vi "uTTA_Calibration_ADC.vi"(6 "AR488_in":refnum<visa-resource-name>, 7 "CommandQueue":refnum<queue>, 8 "error in":errorcluster, 9 "FunctionGen_In":refnum<visa-resource-name>, 10 "DataQueue":refnum<queue>, 11 "TDMS_FileIn":refnum<k34>) -> (0 "error out":errorcluster, 1 "FunctionGen_Out":refnum<visa-resource-name>, 2 "abort":bool, 3 "TDMS_FileOut":refnum<k34>, 4 "AR488_out":refnum<visa-resource-name>)   [LabVIEW 2021]
uses:
  <vilib>/Utility/miscctls.llb/LVPointTypeDef.ctl
  <vilib>/Analysis/6fits.llb/Curve Fitting Criteria.ctl
  eb1c96f3-5bac-4f55-aaa1-37eec1307aa8.vi
  <vilib>/Analysis/NI_AALPro.lvlib
panel:
  out "Voffs Zero Position":dbl
  out "DAC offset":dbl format="%#_6pV"
  out "DAC Residue":dbl caption="Residue" format="%.3p"
  out "DAC slope":dbl format="%#_4pV/Digit"
  in  "START":bool
  out "ADC_Values":dbl[](array[numeric]) format="%#.2g"
  out "ADC_Variance":dbl[](array[numeric]) format="%#.2g"
  out "ADC offset":dbl format="%#_6pV"
  out "ADC lin. res":dbl caption="Residue" format="%.3p"
  out "ADC slope":dbl format="%#_4pV/Digit"
  out "Ref. Setting":u32
  out "ADC Cal.":T1(graph)
  out "PGA setting":u32
  out "Calibration of Channel":u32
  in  "DAC Increments":u32=1000 caption="DAC Voltage\nIncrement" min=1 max=10000 step=1 format="%.3d Counts/Step"
  out "Status":string="Exit"
  in  "abort":bool
  # "1. Connect the function generator with a 50Ohm Terminator and a BNC Y-Adaptor to the input of the uTTA.\n2. Connect a ground lead to the outer Conductor of the BNC line to provide propper grounding\n3. Start the calibration"
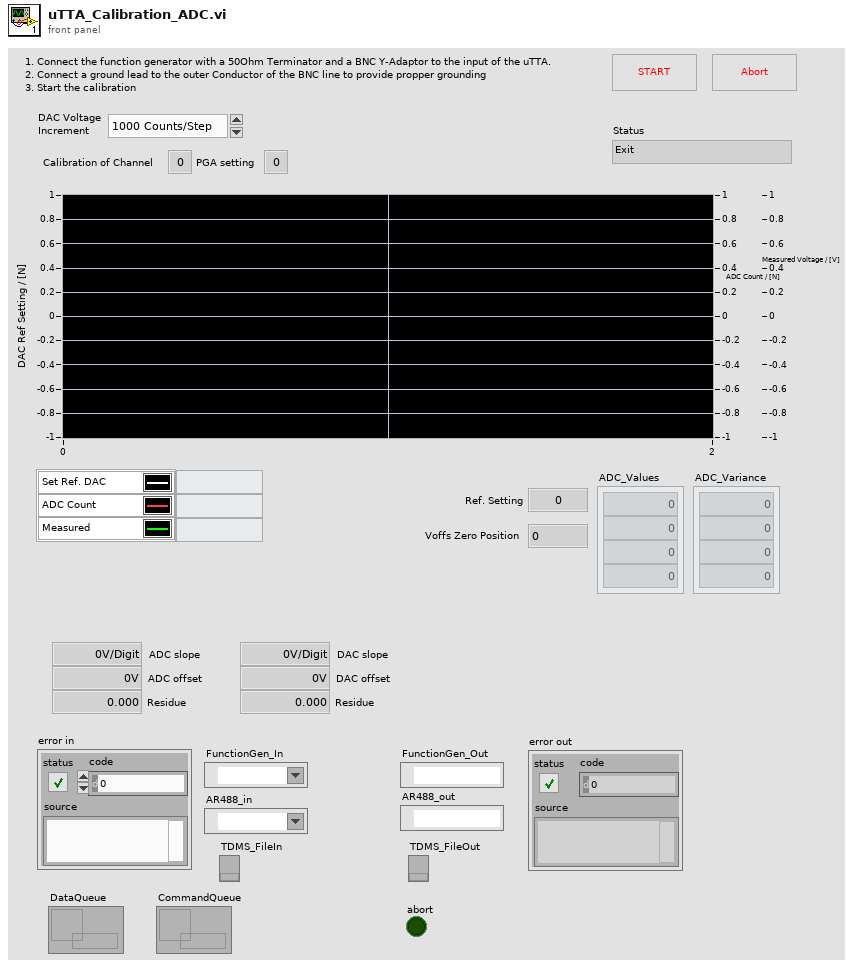
[diagram p1: front panel]
types:
  T1 = cluster{"Ref_Voltage":u32, "mean":dbl, "mean":dbl}
  T2 = typedef "LVPointTypeDef.ctl" = cluster{"Horizontal":i16, "Vertical":i16}
  T3 = cluster{"Ref_Voltage":u32, "mean":dbl, "mean":dbl}[]
  T4 = typedef "NI_AALPro.lvlib/Curve Fitting Criteria.ctl" = u16
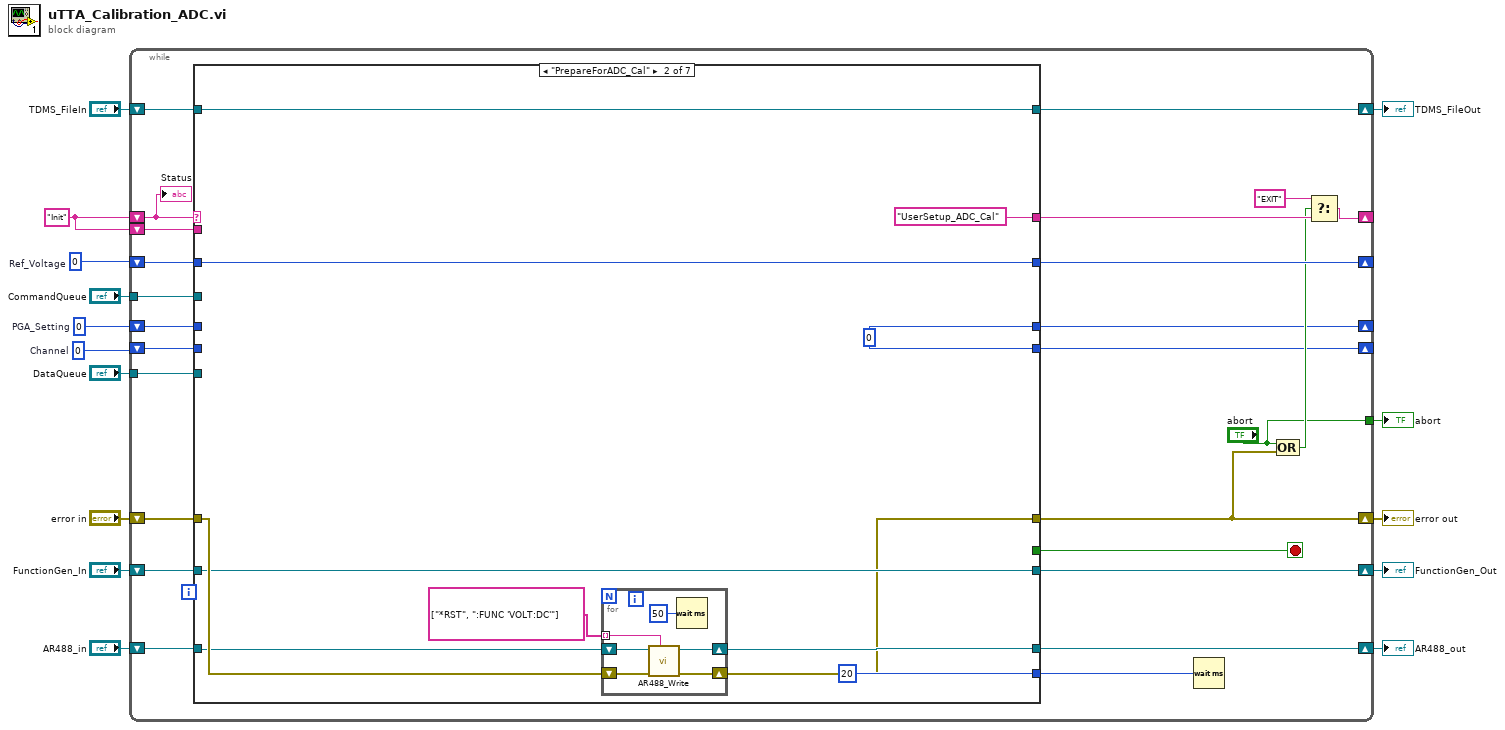
[diagram p0: block diagram]
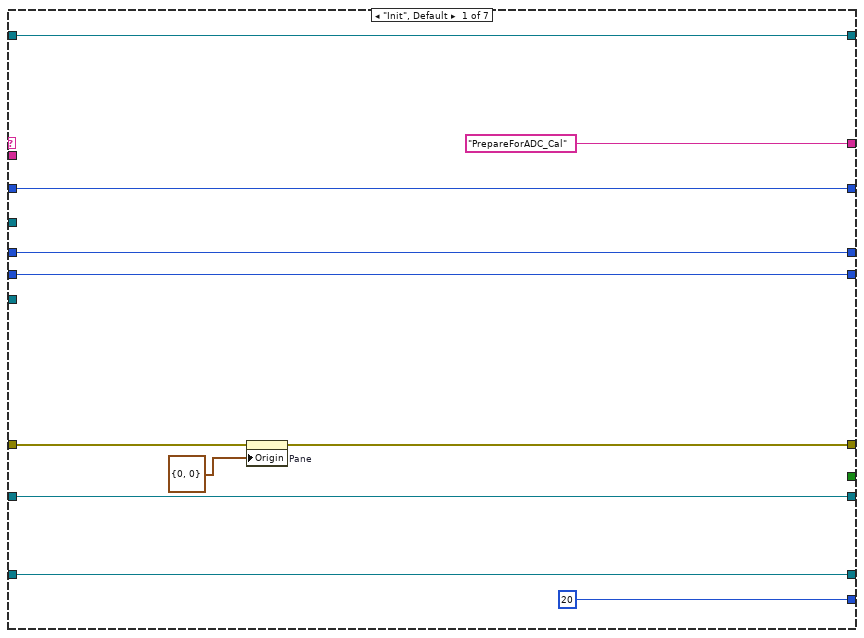
[diagram p2: hidden frame]
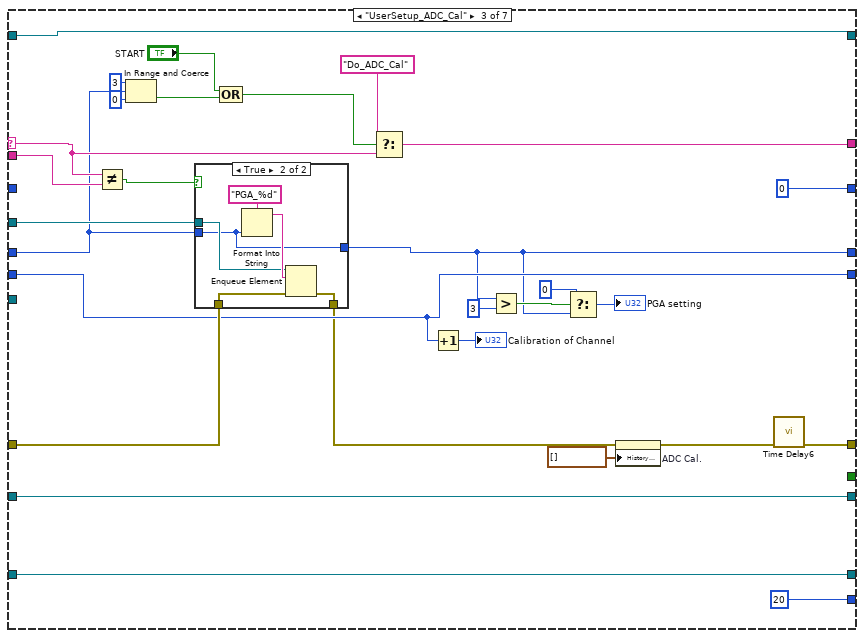
[diagram p3: hidden frame]
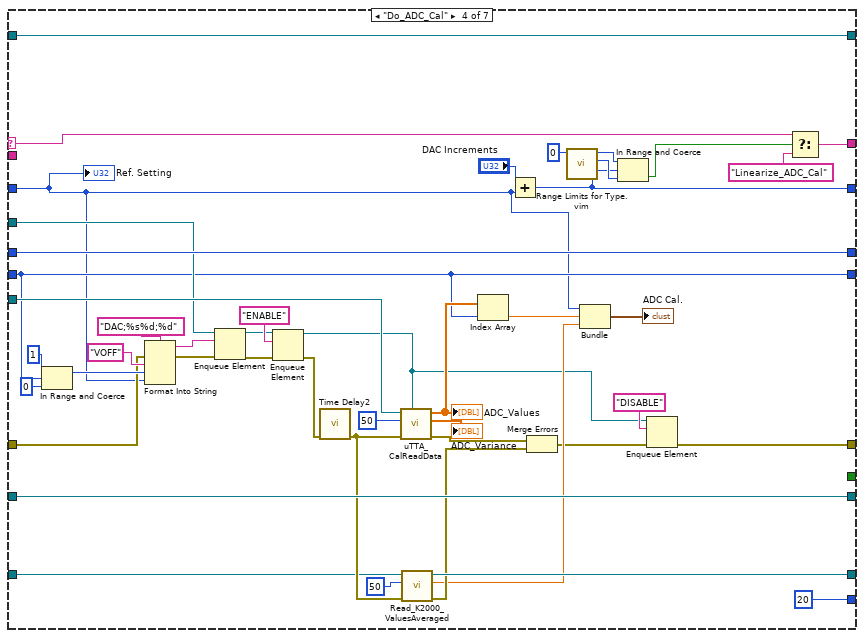
[diagram p5: hidden frame]
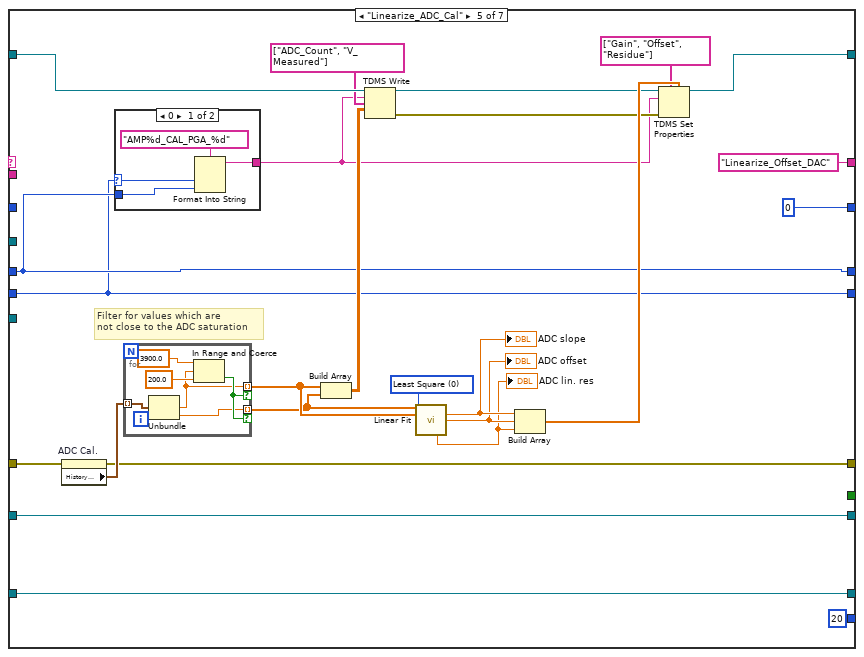
[diagram p6: hidden frame]
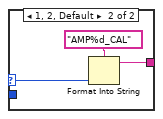
[diagram p7: hidden frame]
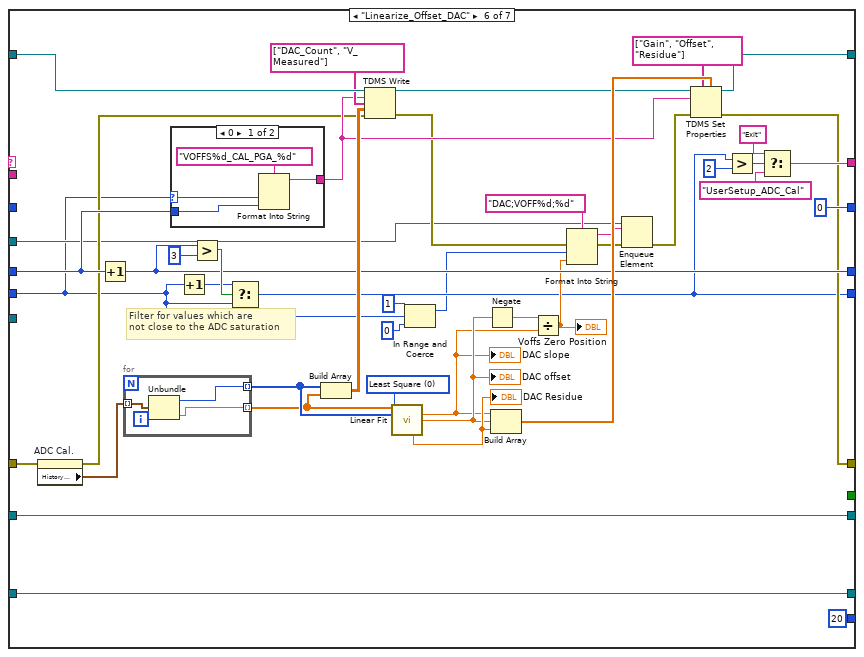
[diagram p8: hidden frame]
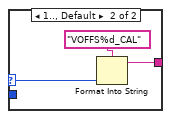
[diagram p9: hidden frame]
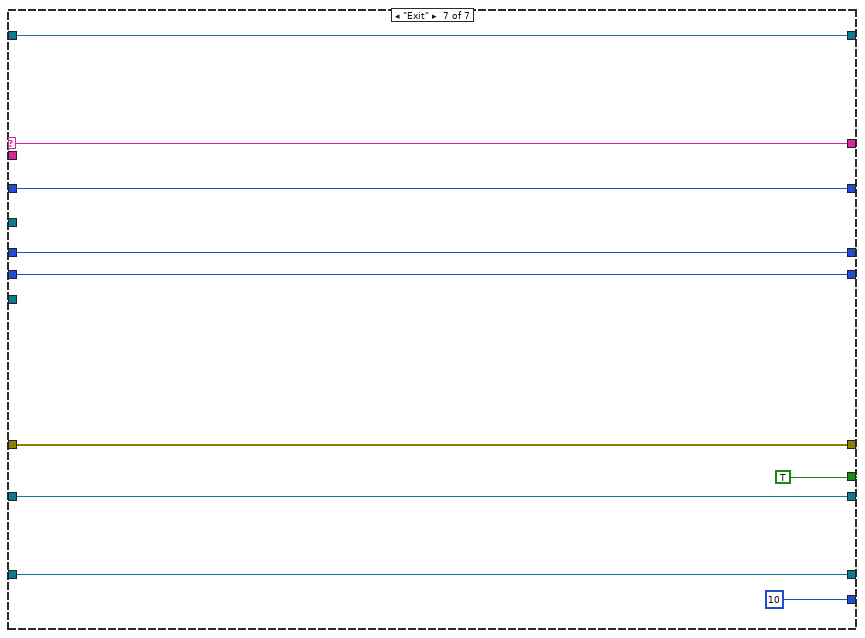
[diagram p10: hidden frame]
diagram:
  w11 = 0  # Channel
  w12 = 0  # PGA_Setting
  w14 = u32 0  # Ref_Voltage
  w13 = "Init"
  n1 = while {
    shift-right: [w27] -> _
    shift-left: w13 -> [w38]
    shift-right: [w25] -> w15
    shift-left: "error in" -> [w40]
    shift-right: [w36] -> w3
    shift-left: "FunctionGen_In" -> [w37]
    shift-right: [w35] -> w2
    shift-left: "AR488_in" -> [w34]
    shift-left: w13 -> [w33]
    tunnel: "CommandQueue" -> [w32]
    tunnel: "DataQueue" -> [w31]
    shift-right: [w29] -> _
    shift-left: w14 -> [w30]
    shift-right: [w22] -> w7
    shift-left: "TDMS_FileIn" -> [w21]
    shift-right: [w19] -> _
    shift-left: w12 -> [w20]
    shift-right: [w17] -> _
    shift-left: w11 -> [w18]
    tunnel: ["abort"] -> w1
    stop <- w23 stop-if-true
    n2 = case shown="\"PrepareForADC_Cal\"" w38 {
      selector: w38 -> [_ _ w81 w147 _ _ w253]
      tunnel: [_ _ _ _ _ _ TRUE] -> w23
      tunnel: w40 -> [w48 w58 w90 w128 w169 w227 w247]
      tunnel: ["PrepareForADC_Cal" ("t") "UserSetup_ADC_Cal" ("t") w97 w146 "Linearize_Offset_DAC" ("t") w208 w253] -> w28
      tunnel: [w44 w52 w72 w107 w155 w195 w247] -> w25
      tunnel: [u32 20 u32 20 u32 20 u32 20 u32 20 u32 20 u32 10] -> w39
      tunnel: w37 -> [w47 w56 w96 w144 w173 w231 w246]
      tunnel: [w47 w56 w96 w144 w173 w231 w246] -> w36
      tunnel: [w46 w53 w95 w117 w171 w229 w245] -> w35
      tunnel: w34 -> [w46 w54 w95 w118 w171 w229 w245]
      tunnel: w33 -> [_ _ w80 _ _ _ _]
      tunnel: w32 -> [_ _ w89 w133 _ w194 _]
      tunnel: w31 -> [_ _ _ w141 _ _ _]
      tunnel: w30 -> [w45 w61 _ w127 _ _ w250]
      tunnel: [w45 w61 u32 0 w121 u32 0 u32 0 w250] -> w29
      tunnel: [w43 w59 w91 w145 w167 w225 w249] -> w22
      tunnel: w21 -> [w43 w59 w91 w145 w168 w226 w249]
      tunnel: w20 -> [w41 _ w76 w143 w158 w211 w244]
      tunnel: [w41 w57 w78 w143 w158 w217 w244] -> w19
      tunnel: w18 -> [w42 _ w85 w132 w156 w189 w248]
      tunnel: [w42 w57 w85 w132 w156 w191 w248] -> w17
      frame "Init", Default {
        n3 = property on="Pane" class="Pane"(error in=w48, "Origin"=T2 {"Horizontal"=0, "Vertical"=0}) -> (error out=w44:errorcluster)  [unwired: 1 in, 1 out]
      }
      frame "PrepareForADC_Cal" {
        w57 = 0 ("Channel")
        n4 = for {
          tunnel: string[] ["*RST", ":FUNC 'VOLT:DC'"] -> [w67] mode=indexing
          shift-right: [w65] -> w53
          shift-left: w54 -> [w68]
          shift-right: [w64] -> w52
          shift-left: w58 -> [w66]
          n5 = call "AR488_Write.vi"("write"=w67, "error in (no error)"=w66, "VISA Refnum in"=w68) -> ("error out"=w64:errorcluster, "VISA Refnum out"=w65:refnum<visa-resource-name>)  [unwired: 7 in]
          n6 = Wait (ms)(milliseconds to wait=u32 50) -> ()  [unwired: 1 out]
        }
      }
      frame "UserSetup_ADC_Cal" {
        n7 = Not Equal?(x=w81, y=w80) -> (x != y?=w79:bool)
        n8 = In Range and Coerce(upper limit=u32 3, x=w76, lower limit=u32 0) -> (In Range?=w82:bool)  [unwired: 1 out]
        n9 = case shown="True" w79 {
          tunnel: w90 -> [w99 w105]
          tunnel: [w99 w104] -> w71
          tunnel: w89 -> [_ w101]
          tunnel: w76 -> [w98 w100]
          tunnel: [w98 w100] -> w78
          frame False {
          }
          frame True {
            n10 = Format Into String(format string="PGA_%d" ("element"), w100) -> (resulting string=w102:string)  [unwired: 2 in, 1 out]
            n11 = Enqueue Element(queue=w101, element=w102, error in (no error)=w105) -> (error out=w104:errorcluster)  [unwired: 1 in, 2 out]
          }
        }
        n12 = Compound Arithmetic op=OR("START", w82) -> (w84:bool)
        n13 = Select(t="Do_ADC_Cal", s=w84, f=w81) -> (s? t:f=w97:string)
        n14 = Increment(x=w85) -> (x+1=→"Calibration of Channel":i32)
        n15 = Greater?(x=w78, y=u32 3) -> (0:w87:bool)
        n16 = Select(t=u32 0, s=w87, f=w78) -> (s? t:f=→"PGA setting":u32)
        n17 = property on="ADC Cal." class="WFChart (strict)"(error in=w71, "History Data"=T3 []) -> (error out=w70:errorcluster)  [unwired: 1 in, 1 out]
        n18 = call "Time Delay6"("error in (no error)"=w70) -> ("error out"=w72:errorcluster)  [unwired: 10 in]
      }
      frame "Do_ADC_Cal" {
        n19 = In Range and Coerce(upper limit=1, x=w132, lower limit=0) -> (coerced(x)=w131:i32)  [unwired: 1 out]
        n20 = Format Into String(format string="DAC;%s%d;%d" ("element"), error in=w128, "VOFF" ("input 1"), w131, w127) -> (resulting string=w136:string, error out=w134:errorcluster)  [unwired: 1 in]
        n21 = Enqueue Element(queue=w133, element=w136, error in (no error)=w134) -> (queue out=w110:refnum<queue>, error out=w111:errorcluster)  [unwired: 1 in, 1 out]
        n22 = Enqueue Element(queue=w110, element="ENABLE", error in (no error)=w111) -> (queue out=w106:refnum<queue>, error out=w112:errorcluster)  [unwired: 1 in, 1 out]
        n23 = call "Time Delay2"("error in (no error)"=w112) -> ("error out"=w119:errorcluster)  [unwired: 10 in]
        n24 = call "uTTA_CalReadData.vi"("Control Queue"=w106, "error in"=w119, "Averaged Values"=50, "Data Queue in"=w141) -> ("error out"=w115:errorcluster, "ADC_Variance"=→"ADC_Variance":dbl[], "ADC_Values"=w138:dbl[])  [unwired: 3 in, 2 out]
        "ADC_Values" <- w138
        n25 = call "Read_K2000_ValuesAveraged.vi"("error in"=w119, "No. Averaged Values"=50, "VISA Refnum in"=w118) -> ("error out"=w116:errorcluster, "mean"=w114:dbl, "VISA Refnum out"=w117:refnum<visa-resource-name>)  [unwired: 6 in]
        n26 = Index Array(array=w138, index=w132) -> (element=w126:dbl)
        n27 = Add(x="DAC Increments", y=w127) -> (x+y=w121:u32)
        n28 = Merge Errors(w115, w116) -> (w108:errorcluster)
        n29 = call "Range Limits for Type.vim"("type"=u16 0) -> ("minimum value for type"=w123:u16, "maximum value for type"=w124:u16)  [unwired: 9 in]
        n30 = Bundle("Ref_Voltage"=w127, "mean"=w126, "mean"=w114) -> (→"ADC Cal.":T1)  [unwired: 1 in]
        n31 = In Range and Coerce(upper limit=w124, x=w121, lower limit=w123) -> (In Range?=w142:bool)  [unwired: 1 out]
        n32 = Enqueue Element(queue=w106, element="DISABLE", error in (no error)=w108) -> (error out=w107:errorcluster)  [unwired: 1 in, 2 out]
        n33 = Select(t=w147, s=w142, f="Linearize_ADC_Cal") -> (s? t:f=w146:string)
        "Ref. Setting" <- w127
      }
      frame "Linearize_ADC_Cal" {
        w174 = T4 0 items=["Least Square", "Least Absolute Residual", "Bisquare"] ("method")
        # "Filter for values which are \nnot close to the ADC saturation"
        n34 = property on="ADC Cal." class="WFChart (strict)"(error in=w169) -> (error out=w155:errorcluster, "History Data"=w175:T3)  [unwired: 1 in, 1 out]
        n35 = case shown="0" w156 {
          selector: w156 -> [w177 w180]
          tunnel: w158 -> [w176 _]
          tunnel: [w178 w181] -> w157
          frame 0 {
            n36 = Format Into String(format string="AMP%d_CAL_PGA_%d" ("group name in (Untitled)"), w177, w176) -> (resulting string=w178:string)  [unwired: 2 in, 1 out]
          }
          frame 1, 2, Default {
            n37 = Format Into String(format string="AMP%d_CAL" ("group name in (Untitled)"), w180) -> (resulting string=w181:string)  [unwired: 2 in, 1 out]
          }
        }
        n38 = for {
          tunnel: w175 -> [w188] mode=indexing
          tunnel: [w184] -> w152 mode=indexing if=w186
          tunnel: [w183] -> w153 mode=indexing if=w186
          n39 = Unbundle(w188) -> ("mean"=w183:dbl, "mean"=w184:dbl)  [unwired: 1 out]
          n40 = In Range and Coerce(upper limit=3900.0, x=w183, lower limit=200.0 ("y")) -> (In Range?=w186:bool)  [unwired: 1 out]
        }
        n41 = Build Array(w153, w152) -> (w166:dbl[][])
        n42 = TDMS Write(0:w168, 5:w157, 7:string[] ["ADC_Count", "V_Measured"], 9:w166) -> (4:w161:refnum<k34>, 15:w160:errorcluster)  [unwired: 2 in, 2 out]
        n43 = call <vilib>:"Linear Fit.vi"("Y"=w152, "X"=w153, "method"=w174) -> ("slope"=w165:dbl, "intercept"=w164:dbl, "residue"=w154:dbl)  [unwired: 8 in, 2 out]
        "ADC offset" <- w164
        "ADC lin. res" <- w154
        "ADC slope" <- w165
        n44 = Build Array(w165, w164, w154) -> (w163:dbl[])
        n45 = TDMS Set Properties(5:w163, 7:string[] ["Gain", "Offset", "Residue"] ("property names"), 8:w160, 10:w157, 11:w161) -> (3:w167:refnum<k34>)  [unwired: 1 in, 3 out]
      }
      frame "Linearize_Offset_DAC" {
        w232 = T4 0 items=["Least Square", "Least Absolute Residual", "Bisquare"] ("method")
        # "Filter for values which are \nnot close to the ADC saturation"
        n46 = property on="ADC Cal." class="WFChart (strict)"(error in=w227) -> (error out=w198:errorcluster, "History Data"=w233:T3)  [unwired: 1 in, 1 out]
        n47 = Increment(x=w211) -> (x+1=w217:i32)
        n48 = for {
          tunnel: w233 -> [w243] mode=indexing
          tunnel: [w241] -> w206 mode=indexing
          tunnel: [w242] -> w207 mode=indexing
          n49 = Unbundle(w243) -> ("Ref_Voltage"=w242:u32, "mean"=w241:dbl)  [unwired: 1 out]
        }
        n50 = case shown="0" w189 {
          selector: w189 -> [w235 w238]
          tunnel: w211 -> [w234 _]
          tunnel: [w236 w239] -> w210
          frame 0 {
            n51 = Format Into String(format string="VOFFS%d_CAL_PGA_%d" ("group name in (Untitled)"), w235, w234) -> (resulting string=w236:string)  [unwired: 2 in, 1 out]
          }
          frame 1.., Default {
            n52 = Format Into String(format string="VOFFS%d_CAL" ("group name in (Untitled)"), w238) -> (resulting string=w239:string)  [unwired: 2 in, 1 out]
          }
        }
        n53 = Increment(x=w189) -> (x+1=w218:i32)
        n54 = Greater?(x=w217, y=u32 3) -> (0:w219:bool)
        n55 = Select(t=w218, s=w219, f=w189) -> (s? t:f=w191:i32)
        n56 = Build Array(w207, w206) -> (w224:dbl[][])
        n57 = TDMS Write(0:w226, 5:w210, 7:string[] ["DAC_Count", "V_Measured"], 9:w224, 11:w198) -> (4:w213:refnum<k34>, 15:w197:errorcluster)  [unwired: 1 in, 2 out]
        n58 = call <vilib>:"Linear Fit.vi"("Y"=w206, "X"=w207, "method"=w232) -> ("slope"=w203:dbl, "intercept"=w204:dbl, "residue"=w209:dbl)  [unwired: 8 in, 2 out]
        "DAC offset" <- w204
        "DAC Residue" <- w209
        "DAC slope" <- w203
        n59 = In Range and Coerce(upper limit=1, x=w189, lower limit=0) -> (coerced(x)=w190:i32)  [unwired: 1 out]
        n60 = Negate(x=w204) -> (-x=w205:dbl)
        n61 = Build Array(w203, w204, w209) -> (w223:dbl[])
        n62 = Divide(x=w205, y=w203) -> (x/y=w199:dbl)
        "Voffs Zero Position" <- w199
        n63 = Format Into String(format string="DAC;VOFF%d;%d" ("element"), error in=w197, w190, w199) -> (resulting string=w202:string, error out=w201:errorcluster)  [unwired: 1 in]
        n64 = Enqueue Element(queue=w194, element=w202, error in (no error)=w201) -> (error out=w196:errorcluster)  [unwired: 1 in, 2 out]
        n65 = TDMS Set Properties(5:w223, 7:string[] ["Gain", "Offset", "Residue"] ("property names"), 8:w196, 10:w210, 11:w213) -> (0:w195:errorcluster, 3:w225:refnum<k34>)  [unwired: 1 in, 2 out]
        n66 = Greater?(x=w191, y=u32 2) -> (0:w215:bool)
        n67 = Select(t="Exit", s=w215, f="UserSetup_ADC_Cal" ("t")) -> (s? t:f=w208:string)
      }
      frame "Exit" {
      }
    }
    n68 = Wait (ms)(milliseconds to wait=w39) -> ()  [unwired: 1 out]
    n69 = Compound Arithmetic op=OR("abort", w25) -> (w24:bool)
    n70 = Select(t="EXIT", s=w24, f=w28) -> (s? t:f=w27:string)
    "Status" <- w38
  }
  "TDMS_FileOut" <- w7
  "error out" <- w15
  "FunctionGen_Out" <- w3
  "AR488_out" <- w2
  "abort" <- w1
